vi "Close_WeatherStation_Connection.vi"() -> (0 "Status/Error string":string)   [LabVIEW 2012]
uses:
  Globals/USB_WeatherLink_Serialnumber.vi
  VantagePro.dll
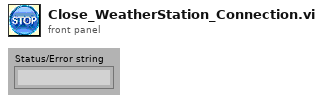
[diagram p1: front panel]
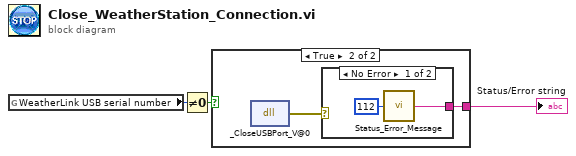
[diagram p0: block diagram]
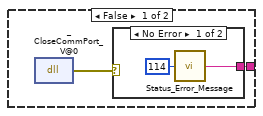
[diagram p2: hidden frame]
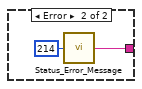
[diagram p3: hidden frame]
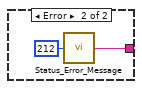
[diagram p4: hidden frame]
diagram:
  n1 = global read "USB_WeatherLink_Serialnumber.vi" "WeatherLink USB serial number"() -> (w2:u32)
  n2 = Not Equal To 0?(x=w2) -> (x != 0?=w1:bool)
  n3 = case shown="True" w1 {
    tunnel: [w4 w10] -> w3
    frame False {
      n4 = dll-call lib="C:/Users/Bob van Eijk/Desktop/LabView Projects 12/HiSPARC Weather Station/VantagePro.dll" fn="_CloseCommPort_V@0" label="Close Serial Port"() -> (error out=w5:errorcluster)  [unwired: 3 in, 2 out]
      n5 = case shown="No Error" w5 {
        tunnel: [w6 w8] -> w4
        frame No Error {
          n6 = call "Status_Error_Message.vi"("Message number"=114) -> ("Status/Error string"=w6:string)
        }
        frame Error {
          n7 = call "Status_Error_Message.vi"("Message number"=214) -> ("Status/Error string"=w8:string)
        }
      }
    }
    frame True {
      n8 = dll-call lib="C:/Users/Bob van Eijk/Desktop/LabView Projects 12/HiSPARC Weather Station/VantagePro.dll" fn="_CloseUSBPort_V@0" label="Close USB Port"() -> (error out=w11:errorcluster)  [unwired: 3 in, 2 out]
      n9 = case shown="No Error" w11 {
        tunnel: [w12 w14] -> w10
        frame No Error {
          n10 = call "Status_Error_Message.vi"("Message number"=112) -> ("Status/Error string"=w12:string)
        }
        frame Error {
          n11 = call "Status_Error_Message.vi"("Message number"=212) -> ("Status/Error string"=w14:string)
        }
      }
    }
  }
  "Status/Error string" <- w3
